vi "Find Update.vi"(8 "Error In":errorcluster, 9 "Current Version":dbl format="%_4g", 11 "search path":path=path "\\\\Nirvana\\AE-General/Cullen Clark") -> (0 "Error Out":errorcluster, 1 "file not found":bool, 2 "newer version?":bool, 3 "update path":path)   [LabVIEW 2018]
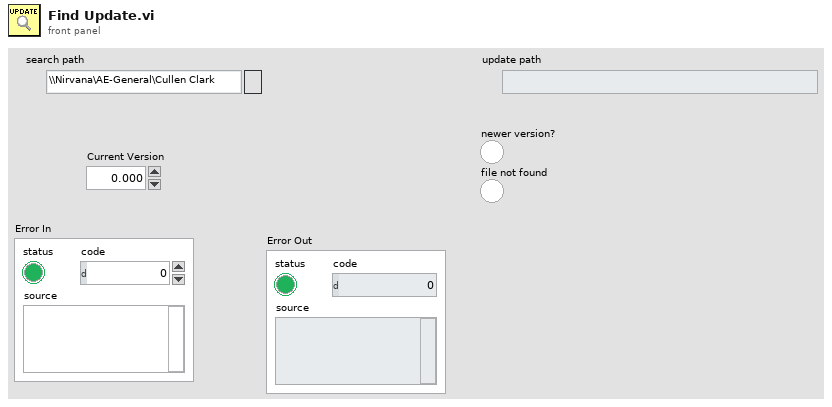
[diagram p1: front panel]
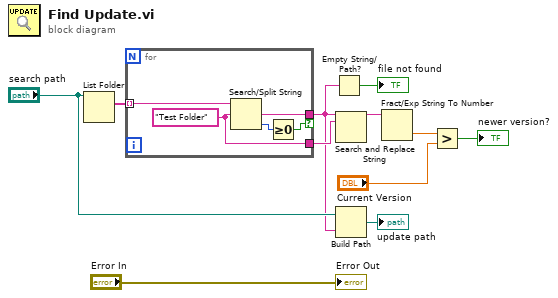
[diagram p0: block diagram]
diagram:
  n1 = List Folder(path="search path") -> (filenames=w11:string[])  [unwired: 3 in, 3 out]
  n2 = for {
    tunnel: w11 -> [w16] mode=indexing
    tunnel: [w15] -> w3 if=w13
    tunnel: [w12] -> w9
    w12 = "Test Folder" ("search string/char (-)")
    n3 = Search/Split String(string=w16, search string/char (-)=w12) -> (match + rest of string=w15:string, offset of match=w14:i32)  [unwired: 1 in, 1 out]
    n4 = Greater Or Equal To 0?(x=w14) -> (x >= 0?=w13:bool)
  }
  n5 = Empty String/Path?(string/path=w3) -> (empty?=→"file not found":bool)
  n6 = Search and Replace String(input string=w3, search string=w9) -> (result string=w10:string)  [unwired: 6 in, 3 out]
  n7 = Build Path(base path="search path", name or relative path=w3) -> (appended path=→"update path":path)
  n8 = Fract/Exp String To Number(string=w10) -> (number=w8:dbl)  [unwired: 3 in, 1 out]
  n9 = Greater?(x=w8, y="Current Version") -> (0:→"newer version?":bool)
  "Error Out" <- "Error In"
